vi "Calibration-Frame9.vi"(11 "Mode in":T1) -> ()   [LabVIEW 2015]
uses:
  Anemometry Sub Vis/Calibration/Calib_mode.ctl
  Anemometry Sub Vis/Globals/Calib_global.vi
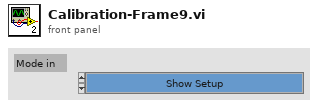
[diagram p1: front panel]
types:
  T1 = typedef "Calib_mode.ctl" = enum16{"Show Setup", "Take a New Calibration Point", "Refit Curve", "Setup Front Panel"}
  T2 = typedef "Cal_Inst_type.ctl" = enum16{"Propeller anemometer", "Pressure Transducer", "Hot wire", "Cross wire velocity", "Cross wire angle", "Generic Linear", "Generic Polynomial", "Generic BackPoly", "Fast FID", "Thermocouple", "Cold wire", "Pulsed Wire"}
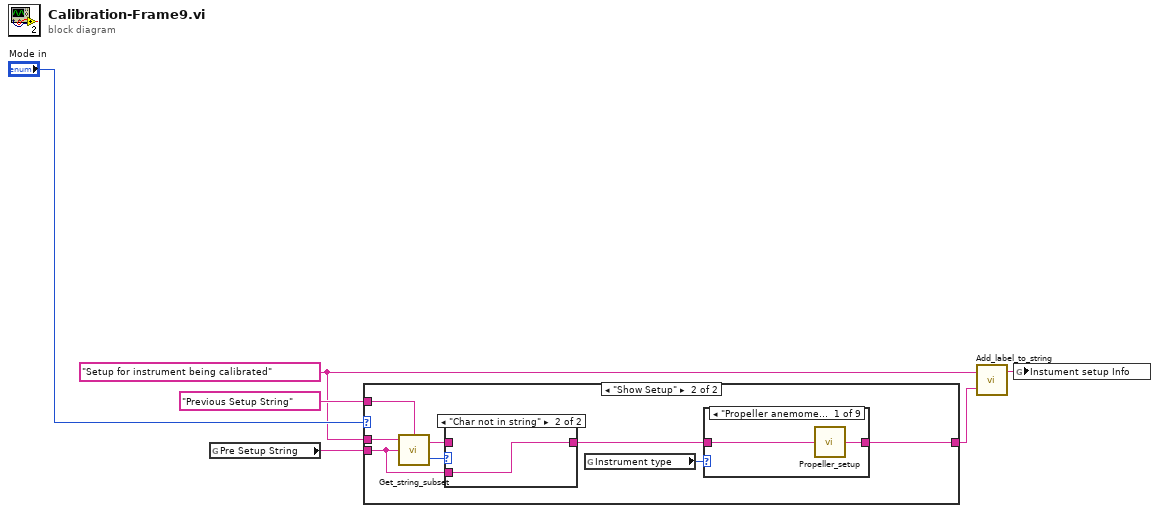
[diagram p0: block diagram]
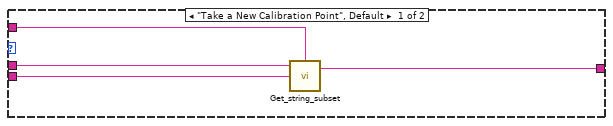
[diagram p2: hidden frame]
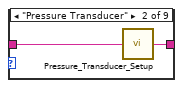
[diagram p4: hidden frame]
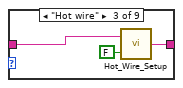
[diagram p5: hidden frame]
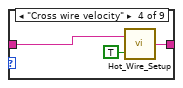
[diagram p6: hidden frame]
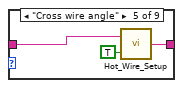
[diagram p7: hidden frame]
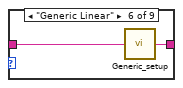
[diagram p8: hidden frame]
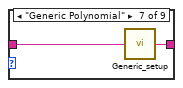
[diagram p9: hidden frame]
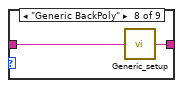
[diagram p10: hidden frame]
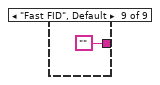
[diagram p11: hidden frame]
diagram:
  w2 = "Setup for instrument being calibrated"
  n1 = global read "Calib_global.vi" "Pre Setup String"() -> (w4:string)
  n2 = case shown="\"Show Setup\"" "Mode in" {
    tunnel: w4 -> [w10 w14]
    tunnel: w2 -> [w9 w13]
    tunnel: [w8 w12] -> w3
    tunnel: "Previous Setup String" ("String Name") -> [w7 w11]
    frame "Take a New Calibration Point", Default {
      n3 = call "Get_string_subset.vi"("String Name"=w7, "String to split"=w10, "File Label"=w9) -> ("Output string"=w8:string)  [unwired: 1 in, 1 out]
    }
    frame "Show Setup" {
      n4 = call "Get_string_subset.vi"("String Name"=w11, "String to split"=w14, "File Label"=w13) -> ("Status"=w16:enum16{"Char in string", "Char not in string"}, "Output string"=w17:string)  [unwired: 1 in]
      n5 = case shown="\"Char not in string\"" w16 {
        tunnel: [w19 w20] -> w15
        tunnel: w17 -> [w19 _]
        tunnel: w14 -> [_ w20]
        frame "Char in string" {
        }
        frame "Char not in string" {
        }
      }
      n6 = global read "Calib_global.vi" "Instrument type"() -> (w18:T2)
      n7 = case shown="\"Propeller anemometer\"" w18 {
        tunnel: [w22 w24 w27 w30 w33 w35 w37 w39 ""] -> w12
        tunnel: w15 -> [w21 w23 w25 w28 w31 w34 w36 w38 _]
        frame "Propeller anemometer" {
          n8 = call "Propeller_setup.vi"("Setup String"=w21) -> ("Output string"=w22:string)
        }
        frame "Pressure Transducer" {
          n9 = call "Pressure_Transducer_Setup.vi"("Setup String"=w23) -> ("Output string"=w24:string)
        }
        frame "Hot wire" {
          n10 = call "Hot_Wire_Setup.vi"("XW?"=FALSE, "Setup String"=w25) -> ("Output string"=w27:string)
        }
        frame "Cross wire velocity" {
          n11 = call "Hot_Wire_Setup.vi"("XW?"=TRUE, "Setup String"=w28) -> ("Output string"=w30:string)
        }
        frame "Cross wire angle" {
          n12 = call "Hot_Wire_Setup.vi"("XW?"=TRUE, "Setup String"=w31) -> ("Output string"=w33:string)
        }
        frame "Generic Linear" {
          n13 = call "Generic_setup.vi"("Setup String"=w34) -> ("Output String"=w35:string)
        }
        frame "Generic Polynomial" {
          n14 = call "Generic_setup.vi"("Setup String"=w36) -> ("Output String"=w37:string)
        }
        frame "Generic BackPoly" {
          n15 = call "Generic_setup.vi"("Setup String"=w38) -> ("Output String"=w39:string)
        }
        frame "Fast FID", Default {
        }
      }
    }
  }
  n16 = call "Add_label_to_string.vi"("String to write"=w3, "File Label"=w2) -> ("Output string"=w1:string)
  n17 = global write "Calib_global.vi" "Instument setup Info"(w1) -> ()
